vi "Compass Plot.vi"() -> ()   [LabVIEW 2023]
doc: "This VI shows how to use the Compass Plot indicator."
uses:
  <vilib>/Math Plots/2D Math Plots/2D Compass/2D Compass XCtrl/2D Compass.xctl
  <vilib>/Math Plots/2D Math Plots/2D Compass/2D Compass Datatype/Public/Plot Helper (Complex).vi
  <vilib>/Math Plots/2D Math Plots/2D Compass/2D Compass Datatype/Public/Plot Helper (Vector).vi
  <vilib>/Math Plots/2D Math Plots/2D Compass/2D Compass Datatype/2D Compass Datatype.lvclass
panel:
  out "Compass Plot (Complex Input)":refnum<class "2D Plot Datatype.lvclass">[](xcontrol)
  out "Compass Plot (Vector Input)":refnum<class "2D Plot Datatype.lvclass">[](xcontrol)
  # "Overview: Demonstrates the Compass Plot indicator.\nInstructions:\nRun the VI."
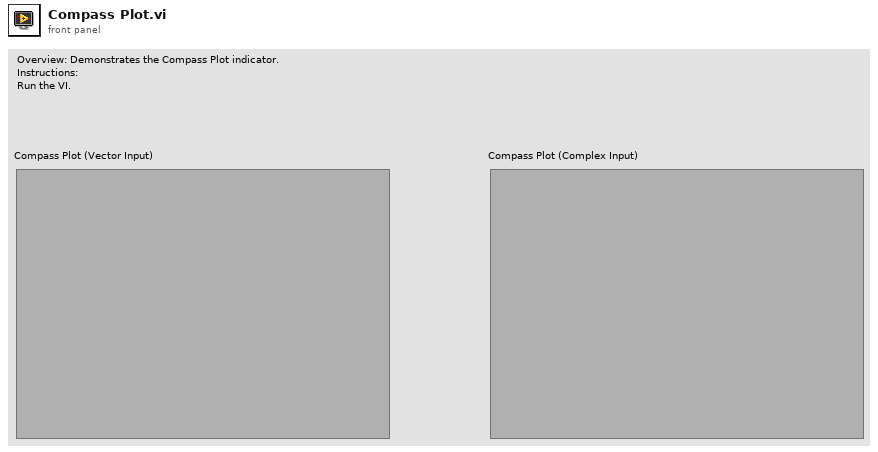
[diagram p1: front panel]
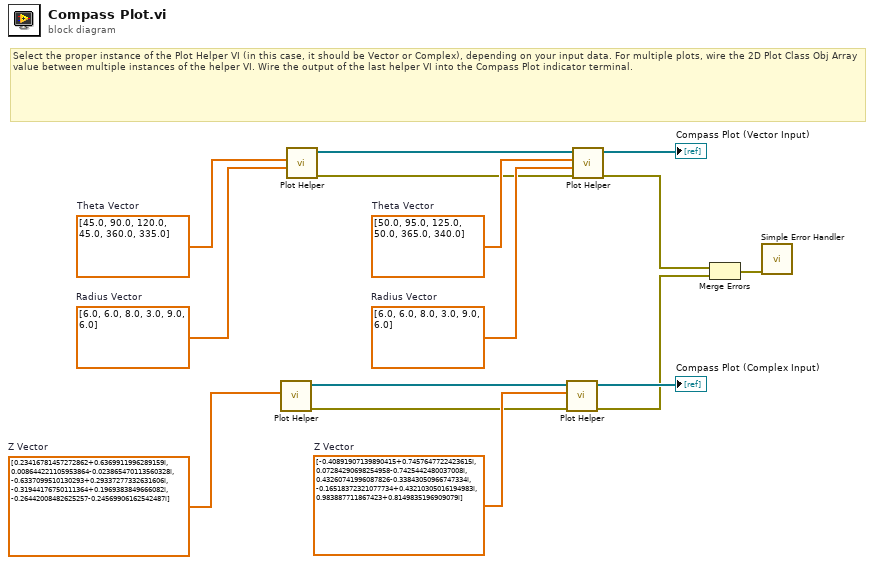
[diagram p0: block diagram]
diagram:
  w8 = dbl[] [6.0, 6.0, 8.0, 3.0, 9.0, 6.0]  # Radius Vector
  w9 = dbl[] [50.0, 95.0, 125.0, 50.0, 365.0, 340.0]  # Theta Vector
  w11 = dbl[] [6.0, 6.0, 8.0, 3.0, 9.0, 6.0]  # Radius Vector
  w12 = dbl[] [45.0, 90.0, 120.0, 45.0, 360.0, 335.0]  # Theta Vector
  w14 = cdb[] [-0.40891907139890415+0.7457647722423615i, 0.07284290698254958-0.7425442480037008i, 0.43260741996087826-0.33843050966747334i, -0.16518372321077734+0.43210305016194983i, 0.983887711867423+0.8149835196909079i]  # Z Vector
  w13 = cdb[] [0.23416781457272862+0.6369911996289159i, 0.008644221105953864-0.023865470113560328i, -0.6337099510130293+0.29337277332631606i, -0.31944176750111364+0.1969383849666082i, -0.26442008482625257-0.24569906162542487i]  # Z Vector
  # "Select the proper instance of the Plot Helper VI (in this case, it should be Vector or Complex), depending on your input data. For multiple plots, wire the 2D Plot Class Obj Array value between multiple instances of the helper VI. Wire the output of the last helper VI into the Compass Plot indicator terminal."
  n1 = call-poly <vilib>:"Plot Helper.vi"("z vector"=w13) -> ("error out"=w4:errorcluster, "2D Plot Class Obj Array out"=w15:refnum<class "2D Plot Datatype.lvclass">[])  [unwired: 2 in, 7 out]
  n2 = call-poly <vilib>:"Plot Helper.vi"("radius vector"=w11, "theta vector"=w12) -> ("error out"=w5:errorcluster, "2D Plot Class Obj Array out"=w10:refnum<class "2D Plot Datatype.lvclass">[])  [unwired: 2 in, 6 out]
  n3 = call-poly <vilib>:"Plot Helper.vi"("error in (no error)"=w4, "z vector"=w14, "2D Plot Class Obj Array in"=w15) -> ("error out"=w2:errorcluster, "2D Plot Class Obj Array out"=→"Compass Plot (Complex Input)":refnum<class "2D Plot Datatype.lvclass">[])  [unwired: 7 out]
  n4 = call-poly <vilib>:"Plot Helper.vi"("error in (no error)"=w5, "radius vector"=w8, "theta vector"=w9, "2D Plot Class Obj Array in"=w10) -> ("error out"=w3:errorcluster, "2D Plot Class Obj Array out"=→"Compass Plot (Vector Input)":refnum<class "2D Plot Datatype.lvclass">[])  [unwired: 6 out]
  n5 = Merge Errors(w3, w2) -> (w1:errorcluster)
  n6 = call <vilib>:"Simple Error Handler.vi"("error in (no error)"=w1) -> ()  [unwired: 4 in, 5 out]
